vi "SS2 Live_Init Communication.vi"(8 "Error In":errorcluster, 11 "SS2 Live Internal Variables in":T1={"okCFrontPanelDevices Refnum"=refnum, "Device Refnum"=refnum, "Display Image"=refnum, "# Live Images"=0, "relative s"=0.0, "# Image Sets"=0, "Message"="", "Current Image Set"=0, "# Datasets"=0, "Current Dataset"=0, "Live Mode"=FALSE, "Recording Mode"=FALSE, "Record Button"=refnum, "Live Button"=refnum, "SS2 Live Gate Data Q Name"="SS2 Live Gate Data Q", "Discard First Image"=FALSE, "Image Information"={"Save ROI Only"=FALSE, "Left"=0, "Top"=0, "Right"=0, "Bottom"=0, "Use Current ROI"=FALSE}, "Image Binning Options"={"Use Image Binning"=FALSE, "X Bin"=1, "Y Bin"=1}} {"Image Binning Options"."Y Bin" min=1; "Image Binning Options"."X Bin" min=1}) -> (0 "Error Out":errorcluster, 1 "Device Refnum":refnum<k24>, 2 "okCFrontPanelDevices Refnum":refnum<k24>, 3 "SS2 Live Internal Variables out":T1={"okCFrontPanelDevices Refnum"=refnum, "Device Refnum"=refnum, "Display Image"=refnum, "# Live Images"=0, "relative s"=0.0, "# Image Sets"=0, "Message"="", "Current Image Set"=0, "# Datasets"=0, "Current Dataset"=0, "Live Mode"=FALSE, "Recording Mode"=FALSE, "Record Button"=refnum, "Live Button"=refnum, "SS2 Live Gate Data Q Name"="SS2 Live Gate Data Q", "Discard First Image"=FALSE, "Image Information"={"Save ROI Only"=FALSE, "Left"=0, "Top"=0, "Right"=0, "Bottom"=0, "Use Current ROI"=FALSE}, "Image Binning Options"={"Use Image Binning"=FALSE, "X Bin"=1, "Y Bin"=1}} {"Image Binning Options"."Y Bin" min=1; "Image Binning Options"."X Bin" min=1})   [LabVIEW 2019]
uses:
  C:/UCLA Thinkpad Google Drive/LabVIEW 2019 SP1/builds/SS2 Live Distribution/Opal Kelly/C# Wrapper/libFrontPanel-csharp.dll
  Opal Kelly/C# Wrapper/libFrontPanel-csharp.dll
  SS2 Live Internal Variables.ctl
  <vilib>/vision/Image Controls.llb/IMAQ Image.ctl
  SS2 Live_Image ROI Information.ctl
  Phasor/Image Binning Options.ctl
  Opal Kelly/C# Wrapper/okFrontPanelC#Wrapper.lvlib
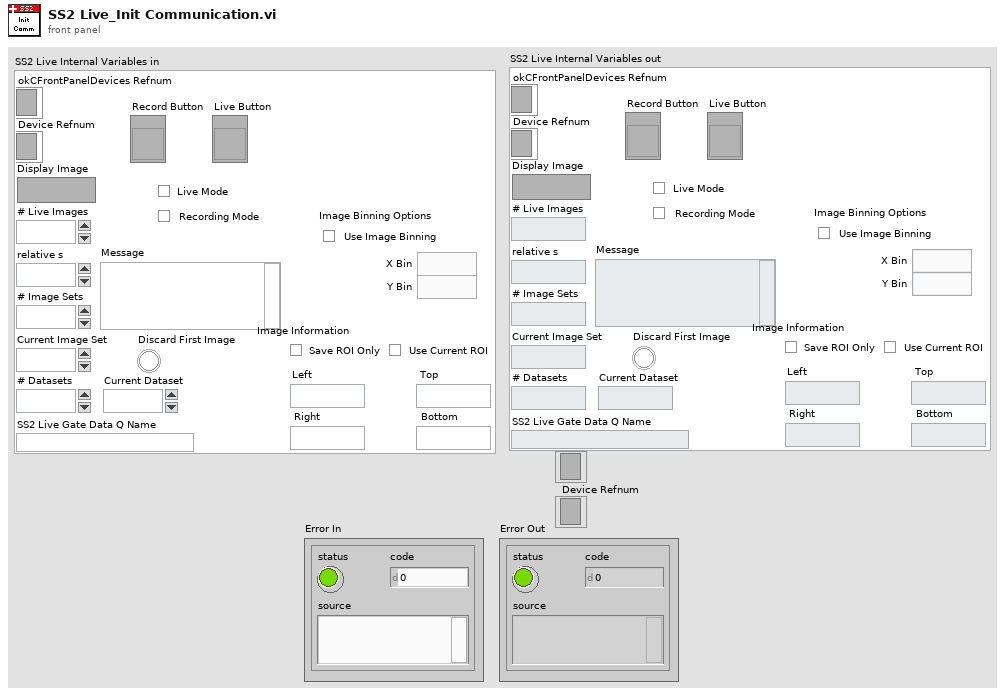
[diagram p1: front panel]
types:
  T1 = typedef "SS2 Live Internal Variables.ctl" = cluster{"okCFrontPanelDevices Refnum":refnum<k24>, "Device Refnum":refnum<k24>, "Display Image":T2, "# Live Images":i32, "relative s":dbl, "# Image Sets":i32, "Message":string, "Current Image Set":i32, "# Datasets":i32, "Current Dataset":i32, "Live Mode":bool, "Recording Mode":bool, "Record Button":refnum<vi>, "Live Button":refnum<vi>, "SS2 Live Gate Data Q Name":string, "Discard First Image":bool, "Image Information":T3, "Image Binning Options":T4}
  T2 = typedef "IMAQ Image.ctl" = refnum<image>
  T3 = typedef "SS2 Live_Image ROI Information.ctl" = cluster{"Save ROI Only":bool, "Left":u16, "Top":u16, "Right":u16, "Bottom":u16, "Use Current ROI":bool}
  T4 = typedef "Image Binning Options.ctl" = cluster{"Use Image Binning":bool, "X Bin":i32, "Y Bin":i32}
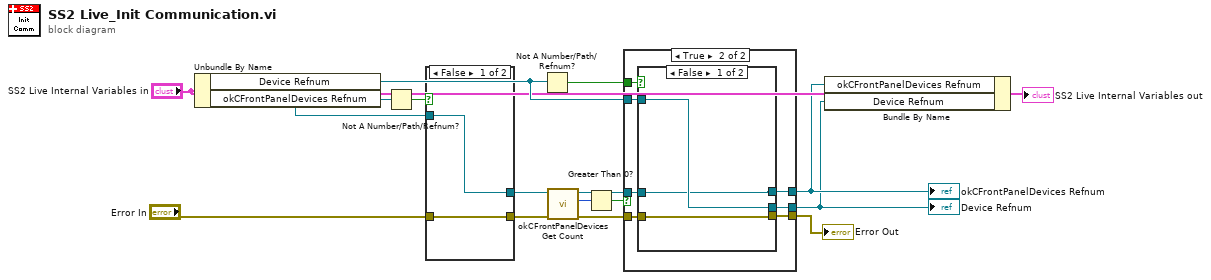
[diagram p0: block diagram]
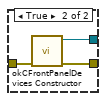
[diagram p2: hidden frame]
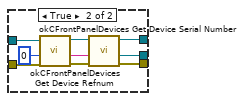
[diagram p4: hidden frame]
diagram:
  n1 = Unbundle By Name("SS2 Live Internal Variables in") -> ("Device Refnum"=w5:refnum<k24>, "okCFrontPanelDevices Refnum"=w7:refnum<k24>)
  n2 = Not A Number/Path/Refnum?(number/path/refnum=w7) -> (NaN/Path/Refnum?=w8:bool)
  n3 = case shown="False" w8 {
    tunnel: [w17 w21] -> w16
    tunnel: [w18 w20] -> w15
    tunnel: "Error In" -> [w17 w19]
    tunnel: w7 -> [w18 _]
    frame False {
    }
    frame True {
      n4 = call "okCFrontPanelDevices Constructor.vi"("Error In"=w19) -> ("Error Out"=w21:errorcluster, "okCFrontPanelDevices Refnum"=w20:refnum<k24>)  [unwired: 9 in]
    }
  }
  n5 = Not A Number/Path/Refnum?(number/path/refnum=w5) -> (NaN/Path/Refnum?=w6:bool)
  n6 = call "okCFrontPanelDevices Get Count.vi"("Error In"=w16, "okCFrontPanelDevices Refnum"=w15) -> ("Error Out"=w11:errorcluster, "GetCount"=w14:i32, "okCFrontPanelDevices Refnum"=w13:refnum<k24>)  [unwired: 7 in]
  n7 = Greater Than 0?(x=w14) -> (x > 0?=w12:bool)
  n8 = case shown="True" w12 {
    tunnel: w13 -> [w23 w30]
    tunnel: w11 -> [w22 w29]
    tunnel: [w23 w28] -> w3
    tunnel: [_ w27] -> w2
    tunnel: [w22 w26] -> w9
    tunnel: w6 -> [_ w25]
    tunnel: w5 -> [_ w24]
    frame False {
    }
    frame True {
      n9 = case shown="False" w25 {
        tunnel: w30 -> [w32 w39]
        tunnel: w29 -> [w31 w38]
        tunnel: [w32 w36] -> w28
        tunnel: [w33 w35] -> w27
        tunnel: [w31 w34] -> w26
        tunnel: w24 -> [w33 _]
        frame False {
        }
        frame True {
          n10 = call "okCFrontPanelDevices Get Device Serial Number.vi"("Error In"=w38, "Device ID"=0, "okCFrontPanelDevices Refnum"=w39) -> ("Error Out"=w41:errorcluster, "Serial Number"=w42:string, "okCFrontPanelDevices Refnum"=w40:refnum<k24>)  [unwired: 6 in]
          n11 = call "okCFrontPanelDevices Get Device Refnum.vi"("Error In"=w41, "Serial Number"=w42, "okCFrontPanelDevices Refnum"=w40) -> ("Error Out"=w34:errorcluster, "Device Refnum"=w35:refnum<k24>, "okCFrontPanelDevices Refnum"=w36:refnum<k24>)  [unwired: 6 in]
        }
      }
    }
  }
  "Error Out" <- w9
  "okCFrontPanelDevices Refnum" <- w3
  "Device Refnum" <- w2
  n12 = Bundle By Name(cluster="SS2 Live Internal Variables in", "okCFrontPanelDevices Refnum"=w3, "Device Refnum"=w2) -> (→"SS2 Live Internal Variables out":T1)
